vi "mouse_position_proof_of_concept.vi"() -> ()   [LabVIEW 2017]
uses:
  <vilib>/Utility/inputDevices.llb/mouseAcquire.vi
panel:
  out "Scroll":string
  out "Buttons":T1
  out "Mouse position relative to 2D picture":cluster{"X":i32, "Y":i32}
  out "Mouse position relative to virtual pane":cluster{"X":i32, "Y":i32}
  out "Window position relative to virtual pane":cluster{"X":i16, "Y":i16}
  out "Pane origin":cluster{"X":i16, "Y":i16}
  out "2D Picture":picture
  out "2D picture position":cluster{"X":i32, "Y":i32}
  out "Window relative to screen":cluster{"X":i16, "Y":i16}
  out "Mouse relative to screen":cluster{"X":i32, "Y":i32}
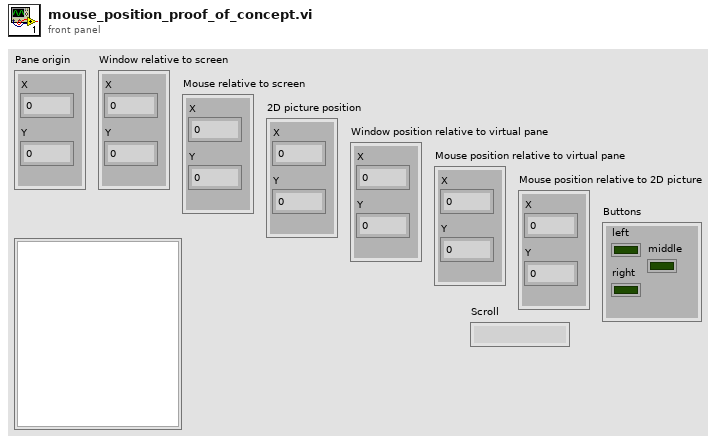
[diagram p1: front panel]
types:
  T1 = cluster{"left":bool, "right":bool, "middle":bool}
  T2 = cluster{"Horizontal":i32, "Vertical":i32, "Scrolling":i32}
  T3 = cluster{"button 1":bool, "button 2":bool, "button 3":bool, "button 4":bool}
  T4 = typedef "LVRectTypeDef.ctl" = cluster{"Left":i16, "Top":i16, "Right":i16, "Bottom":i16}
  T5 = typedef "LVPointTypeDef.ctl" = cluster{"Horizontal":i16, "Vertical":i16}
  T6 = cluster{"button 1":bool, "button 2":bool, "button 3":bool}
  T7 = typedef "LVPositionTypeDef.ctl" = cluster{"Left":i32, "Top":i32}
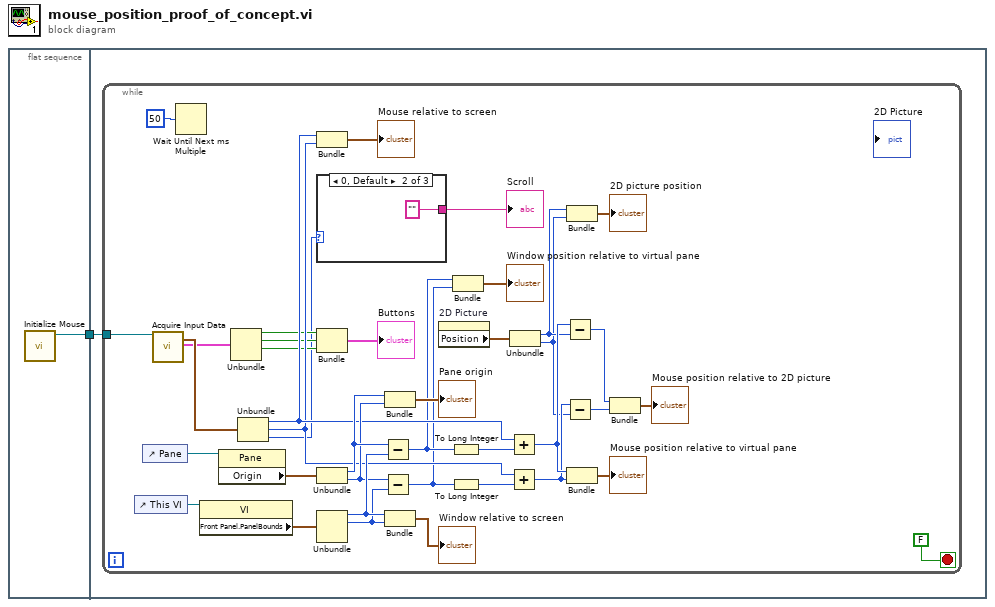
[diagram p0: block diagram]
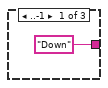
[diagram p2: hidden frame]
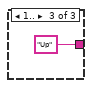
[diagram p3: hidden frame]
diagram:
  n1 = flat-sequence {
    tunnel: [w2] -> w1
    tunnel: w1 -> [w3]
    frame #0 {
      n2 = call <vilib>:"Initialize Mouse.vi"() -> ("device ID"=w2:refnum<k1>)  [unwired: 10 in, 1 out]
    }
    frame #1 {
      n3 = while {
        tunnel: w3 -> [w42]
        stop <- FALSE stop-if-true
        n4 = control-ref of="This VI"() -> (w37:refnum<vi>)
        n5 = control-ref of="Pane"() -> (w32:refnum<vi>)
        n6 = call-poly <vilib>:"Acquire Input Data.vi"("device ID"=w42) -> ("axis info"=w39:T2, "button info"=w10:T3)  [unwired: 15 in, 2 out]
        n7 = Wait Until Next ms Multiple(millisecond multiple=u32 50) -> ()  [unwired: 1 out]
        n8 = property class="VI"(reference=w37) -> ("Front Panel.PanelBounds"=w38:T4)  [unwired: 1 in, 2 out]
        n9 = property class="Pane"(reference=w32) -> ("Origin"=w30:T5)  [unwired: 1 in, 2 out]
        n10 = Unbundle(w10) -> ("button 1"=w8:bool, "button 2"=w7:bool, "button 3"=w6:bool)  [unwired: 1 out]
        n11 = Unbundle(w39) -> ("Horizontal"=w24:i32, "Vertical"=w23:i32, "Scrolling"=w5:i32)
        n12 = Bundle("Horizontal"=w24, "Vertical"=w23) -> (→"Mouse relative to screen":cluster{"Horizontal":i32, "Vertical":i32})  [unwired: 1 in]
        n13 = case shown="0, Default" w5 {
          tunnel: ["Down" "" "Up"] -> w4
          frame ..-1 {
          }
          frame 0, Default {
          }
          frame 1.. {
          }
        }
        "Scroll" <- w4
        n14 = Bundle("button 1"=w8, "button 2"=w7, "button 3"=w6) -> (→"Buttons":T6)  [unwired: 1 in]
        n15 = Unbundle(w30) -> ("Horizontal"=w28:i16, "Vertical"=w26:i16)
        n16 = Unbundle(w38) -> ("Left"=w29:i16, "Top"=w27:i16)  [unwired: 2 out]
        n17 = Subtract(x=w28, y=w29) -> (x-y=w21:i16)
        n18 = Subtract(x=w26, y=w27) -> (x-y=w20:i16)
        n19 = Bundle("Horizontal"=w28, "Vertical"=w26) -> (→"Pane origin":cluster{"Horizontal":i16, "Vertical":i16})  [unwired: 1 in]
        n20 = Bundle("Left"=w29, "Top"=w27) -> (→"Window relative to screen":cluster{"Left":i16, "Top":i16})  [unwired: 1 in]
        n21 = property on="2D Picture" class="Pict"() -> ("Position"=w33:T7)  [unwired: 2 in, 2 out]
        n22 = To Long Integer(number=w21) -> (32bit integer=w22:i32)
        n23 = To Long Integer(number=w20) -> (32bit integer=w19:i32)
        n24 = Bundle(w21, w20) -> (→"Window position relative to virtual pane":cluster{i16, i16})  [unwired: 1 in]
        n25 = Add(x=w24, y=w22) -> (x+y=w17:i32)
        n26 = Add(x=w23, y=w19) -> (x+y=w16:i32)
        n27 = Unbundle(w33) -> ("Left"=w15:i32, "Top"=w14:i32)
        n28 = Subtract(x=w17, y=w15) -> (x-y=w13:i32)
        n29 = Subtract(x=w16, y=w14) -> (x-y=w12:i32)
        n30 = Bundle("Left"=w15, "Top"=w14) -> (→"2D picture position":cluster{"Left":i32, "Top":i32})  [unwired: 1 in]
        n31 = Bundle(w17, w16) -> (→"Mouse position relative to virtual pane":cluster{i32, i32})  [unwired: 1 in]
        n32 = Bundle(w13, w12) -> (→"Mouse position relative to 2D picture":cluster{i32, i32})  [unwired: 1 in]
      }
    }
  }
